vi "未命名 1.vi"(8 "error in (no error)":errorcluster caption="错误输入（无错误）", 11 "模块模板 输入":refnum<class "模块模板.lvclass">) -> (0 "error out":errorcluster caption="错误输出", 3 "模块模板 输出":refnum<class "模块模板.lvclass">)   [LabVIEW 2017]
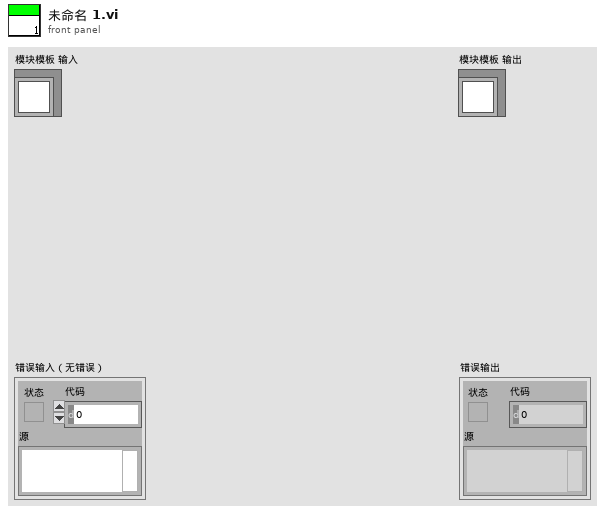
[diagram p1: front panel]
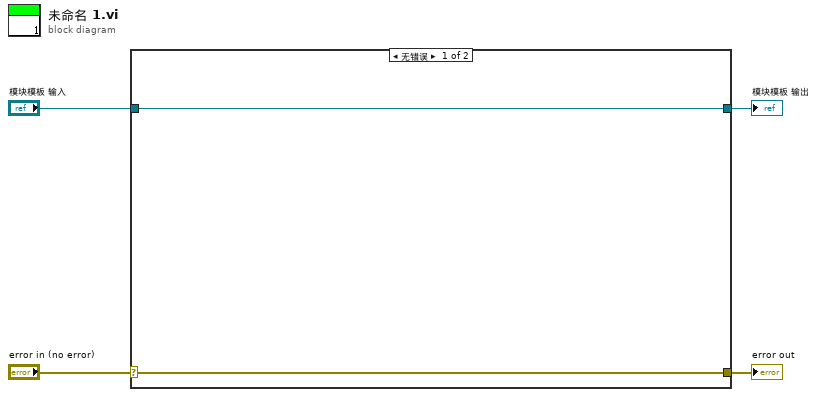
[diagram p0: block diagram]
diagram:
  n1 = case shown="无错误" "error in (no error)" {
    selector: "error in (no error)" -> [w5 w8]
    tunnel: [w5 w8] -> w3
    tunnel: [w6 w7] -> w1
    tunnel: "模块模板 输入" -> [w6 w7]
    frame No Error {
    }
    frame Error {
    }
  }
  "error out" <- w3
  "模块模板 输出" <- w1
